vi "Set Active Window_KT.vi"(11 "hWnd":u32) -> (1 "hWnd active before":u32, 3 "hWnd dup":u32)   [LabVIEW 2017, in "KTools.lvlib"]
doc: "<----Set Active Window----->\nSets given window handle as active window.\nReturns previous window handle which was active."
uses:
  KTools.lvlib
  user32.dll
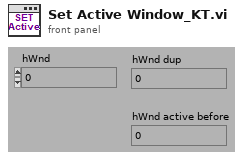
[diagram p1: front panel]
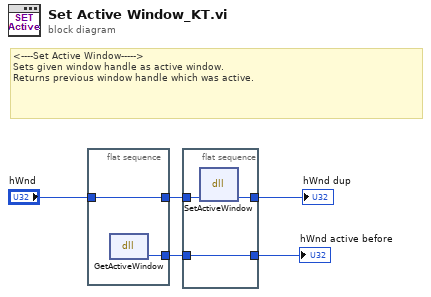
[diagram p0: block diagram]
diagram:
  # "<----Set Active Window----->\nSets given window handle as active window.\nReturns previous window handle which was active."
  n1 = flat-sequence {
    tunnel: [w7] -> w1
    tunnel: [w6] -> w4
    tunnel: "hWnd" -> [w6]
    frame #0 {
      n2 = dll-call lib="user32.dll" fn="GetActiveWindow"() -> ("hWnd"=w7:u32)  [unwired: 3 in, 2 out]
    }
  }
  n3 = flat-sequence {
    tunnel: [w10] -> w5
    tunnel: w4 -> [w9]
    tunnel: [w8] -> w2
    tunnel: w1 -> [w8]
    frame #0 {
      n4 = dll-call lib="user32.dll" fn="SetActiveWindow" ("GetActiveWindow")("hWnd"=w9) -> ("hWnd"=w10:u32)  [unwired: 4 in, 2 out]
    }
  }
  "hWnd dup" <- w5
  "hWnd active before" <- w2
